vi "Initialize Scrollbar.vi"(8 "error in (no error)":errorcluster, 11 "PanelArray in":refnum<class "PanelArray.lvclass">) -> (0 "error out":errorcluster, 3 "PanelArray out":refnum<class "PanelArray.lvclass">)   [LabVIEW 2018, in "OOPanel.lvlib" / "PanelArray.lvclass"]
uses:
  PanelArray.lvclass
  PanelArray.lvclass/PanelArray.ctl
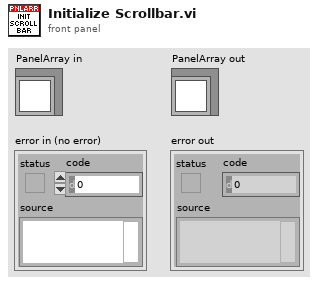
[diagram p1: front panel]
types:
  T1 = typedef "OOPanel.lvlib/PanelArray.lvclass/Ref Data.ctl" = cluster{"State":T2, "Refs":T3, "Events":T4, "Scrolling":T5, "Panels":T6}
  T2 = typedef "OOPanel.lvlib/PanelArray.lvclass/State.ctl" = cluster{"Defer Updates":bool, "Running":bool, "Dynamic Sizing":bool, "Borders":bool}
  T3 = typedef "OOPanel.lvlib/PanelArray.lvclass/Refs.ctl" = cluster{"SubPanels":refnum<vi>[], "Scrollbar":refnum<vi>, "Owning Panel":refnum<vi>}
  T4 = typedef "OOPanel.lvlib/PanelArray.lvclass/Events.ctl" = cluster{"Close":refnum<user-event>}
  T5 = typedef "OOPanel.lvlib/PanelArray.lvclass/Scrolling.ctl" = cluster{"Size":i32, "Max":i32, "Current":i32, "Top Index":i32, "Heights":i32[]}
  T6 = typedef "OOPanel.lvlib/PanelArray.lvclass/Panels.ctl" = cluster{"All":refnum<class "Panel.lvclass">[], "Visible":refnum<class "Panel.lvclass">[], "Blank":refnum<class "ArrayBlank.lvclass">}
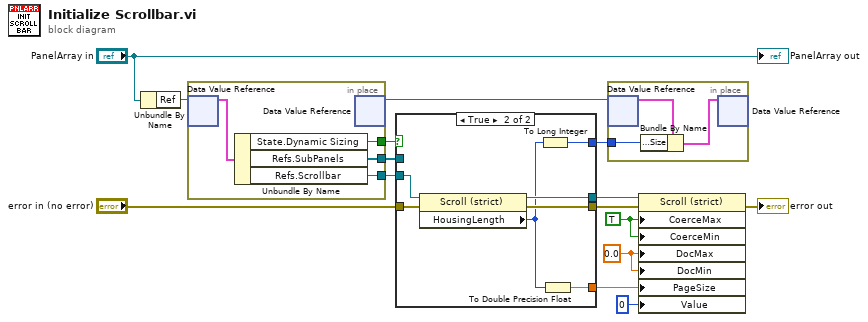
[diagram p0: block diagram]
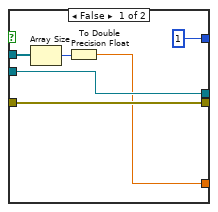
[diagram p2: hidden frame]
diagram:
  w14 = 0.0 ("Doc Max")
  w15 = TRUE ("Coerce Maximum Value")
  n1 = Unbundle By Name("PanelArray in") -> ("Ref"=w6:refnum<data-value>)
  n2 = in-place {
    in-place-border: [w18] -> w3
    in-place-border: [w17] -> w1
    in-place-border: [w16] -> w2
    n3 = in-place-dvr #1(w6) -> (w19:T1)  [unwired: 1 out]
    n4 = Unbundle By Name(w19) -> ("State.Dynamic Sizing"=w18:bool, "Refs.SubPanels"=w17:refnum<vi>[], "Refs.Scrollbar"=w16:refnum<vi>)
    n5 = in-place-dvr #1() -> (w4:refnum<data-value>)  [unwired: 1 in, 1 out]
  }
  n6 = case shown="True" w3 {
    tunnel: "error in (no error)" -> [w24 w32]
    tunnel: [w25 w31] -> w10
    tunnel: [w24 w30] -> w9
    tunnel: [w20 w29] -> w8
    tunnel: [1 w27] -> w7
    tunnel: w2 -> [w25 w26]
    tunnel: w1 -> [w23 _]
    frame False {
      n7 = Array Size(array=w23) -> (size(s)=w21:i32)
      n8 = To Double Precision Float(number=w21) -> (double precision float=w20:dbl)
    }
    frame True {
      n9 = property class="Scroll (strict)"(reference=w26, error in=w32) -> (reference out=w31:refnum<vi>, error out=w30:errorcluster, "HousingLength"=w28:u32)
      n10 = To Long Integer(number=w28) -> (32bit integer=w27:i32)
      n11 = To Double Precision Float(number=w28) -> (double precision float=w29:dbl)
    }
  }
  n12 = in-place {
    in-place-border: w7 -> [w33]
    n13 = in-place-dvr #2(w4) -> (w35:T1)  [unwired: 1 out]
    n14 = Bundle By Name(cluster=w35, "Scrolling.Size"=w33) -> (w34:T1)
    n15 = in-place-dvr #2(w34) -> ()  [unwired: 2 out]
  }
  n16 = property class="Scroll (strict)"(reference=w10, error in=w9, "CoerceMax"=w15, "CoerceMin"=w15, "DocMax"=w14, "DocMin"=w14, "PageSize"=w8, "Value"=0) -> (error out=→"error out":errorcluster)  [unwired: 1 out]
  "PanelArray out" <- "PanelArray in"
